vi "Update PID Parameters.vi"(8 "error in (no error)":errorcluster, 10 "PID Settings":refnum<vi>, 11 "Item Ref in":T1 format="%.0x") -> (0 "error out":errorcluster, 3 "Item Ref out":T1=18446744073709551615 format="%.0x")   [LabVIEW 2019, in "Control Addon System Explorer.lvlib"]
uses:
  Control Addon System Explorer.lvlib
  <vilib>/NI VeriStand/Custom Device API/Custom Device Item Ref.ctl
  Types/Action.ctl
  Addon Shared/SubVIs/Constants.vi
  <vilib>/NI VeriStand/Custom Device API/NI VeriStand - Get Item Property.vi
  <vilib>/NI VeriStand/Custom Device API/Get Item Property (Boolean).vi
  <vilib>/NI VeriStand/Custom Device API/Get Item Property (String).vi
  <vilib>/NI VeriStand/Custom Device API/NI VeriStand - Set Item Property.vi
  <vilib>/NI VeriStand/Custom Device API/Set Item Property (Boolean).vi
  <vilib>/NI VeriStand/Custom Device API/Set Item Property (String).vi
  <vilib>/NI VeriStand/Custom Device API/Custom Device API.lvlib
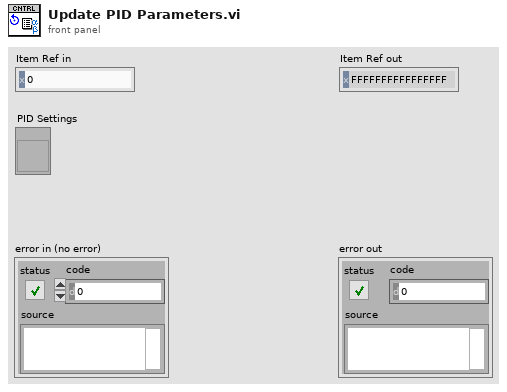
[diagram p1: front panel]
types:
  T1 = typedef "Custom Device API.lvlib/Custom Device Item Ref.ctl" = u64
  T2 = typedef "Control Addon System Explorer.lvlib/Action.ctl" = enum16{"Get", "Set"}
  T3 = typedef "Control Addon Shared.lvlib/PID Parameters.ctl" = cluster{"Enable Live Updates":bool, "Enable Gain Scheduling":bool, "PID Parameters":dbl[][]}
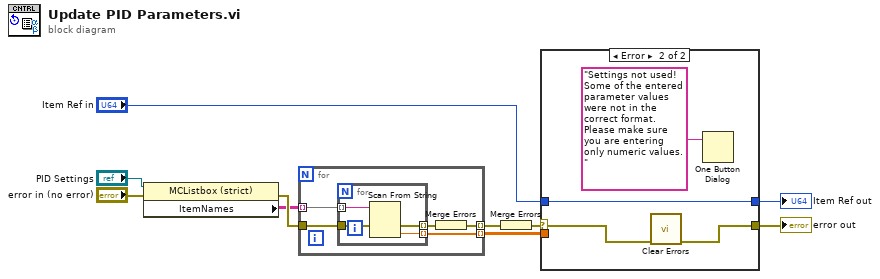
[diagram p0: block diagram]
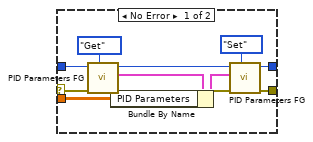
[diagram p2: hidden frame]
diagram:
  n1 = property class="MCListbox (strict)"(reference="PID Settings", error in="error in (no error)") -> (error out=w10:errorcluster, "ItemNames"=w5:string[][])  [unwired: 1 out]
  n2 = for {
    tunnel: w5 -> [w15] mode=indexing
    tunnel: [w14] -> w2 mode=indexing
    tunnel: [w13] -> w6 mode=indexing
    tunnel: w10 -> [w11]
    n3 = for {
      tunnel: w15 -> [w19] mode=indexing
      tunnel: [w18] -> w14 mode=indexing
      tunnel: [w17] -> w12 mode=indexing
      tunnel: w11 -> [w16]
      n4 = Scan From String(input string=w19, error in=w16) -> (error out=w17:errorcluster, output 1=w18:dbl)  [unwired: 3 in, 2 out]
    }
    n5 = Merge Errors(w12) -> (w13:errorcluster)
  }
  n6 = Merge Errors(w6) -> (w7:errorcluster)
  n7 = case shown="Error" w7 {
    selector: w7 -> [w29 w34]
    tunnel: "Item Ref in" -> [w25 w33]
    tunnel: [w24 w31] -> w9
    tunnel: w2 -> [w21 _]
    tunnel: [w20 w33] -> w1
    frame No Error {
      n8 = call "PID Parameters FG.vi"("Action"=Action."Get", "error in (no error)"=w29, "Node Ptr"=w25) -> ("error out"=w27:errorcluster, "Parameters"=w23:T3, "Item Ref out"=w26:T1)  [unwired: 6 in]
      n9 = Bundle By Name(cluster=w23, "PID Parameters"=w21) -> (w22:T3)
      n10 = call "PID Parameters FG.vi"("Action"=Action."Set", "error in (no error)"=w27, "Parameters"=w22, "Node Ptr"=w26) -> ("error out"=w24:errorcluster, "Item Ref out"=w20:T1)  [unwired: 5 in, 1 out]
    }
    frame Error {
      n11 = call <vilib>:"Clear Errors.vi"("error in (no error)"=w34) -> ("error out"=w31:errorcluster)  [unwired: 5 in, 1 out]
      n12 = One Button Dialog(message="Settings not used!  Some of the entered parameter values were not in the correct format.  Please make sure you are entering only numeric values.") -> ()  [unwired: 1 in, 1 out]
    }
  }
  "error out" <- w9
  "Item Ref out" <- w1
